vi "Replicate Core.vi"(7 "subchannel":i32, 9 "# event structures":u16=2, 10 "element (unused)":cluster{"cmd":string, "data":variant}, 11 "data in":refnum<class "EventMessengerMData.lvclass">) -> (2 "event registration refnums":refnum<event-registration>[](array[refnum]), 3 "data out":refnum<class "EventMessengerMData.lvclass">)   [LabVIEW 2019, in "Event MessengerM.lvlib" / "EventMessengerMData.lvclass"]
uses:
  EventMessengerMData.lvclass
  EventMessengerMData.lvclass/EventMessengerMData.ctl
  Event Data.ctl
  Event MessengerM.lvlib
  <vilib>/Utility/miscctls.llb/LVMapReplaceAction.ctl
panel:
  # "See note on block diagram."
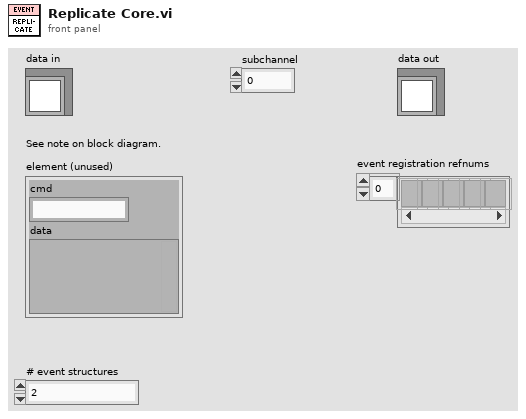
[diagram p1: front panel]
types:
  T1 = typedef "LVMapReplaceAction.ctl" = enum32{"Modify Entry only if found", "Add or Modify Entry", "Delete Entry"}
  T2 = typedef "Event MessengerM.lvlib/Event Data.ctl" = cluster{"msg":cluster{"cmd":string, "data":variant}, "valid?":bool, "last?":bool, "aborted?":bool}
  T3 = map{i32, cluster{"Write Count":u32, "Reg Refnum":u32, "aborted?":bool, "last element?":bool, "Event Refnum":refnum<user-event>}}
  T4 = cluster{"Write Count":u32, "Reg Refnum":u32, "aborted?":bool, "last element?":bool, "Event Refnum":refnum<user-event>}
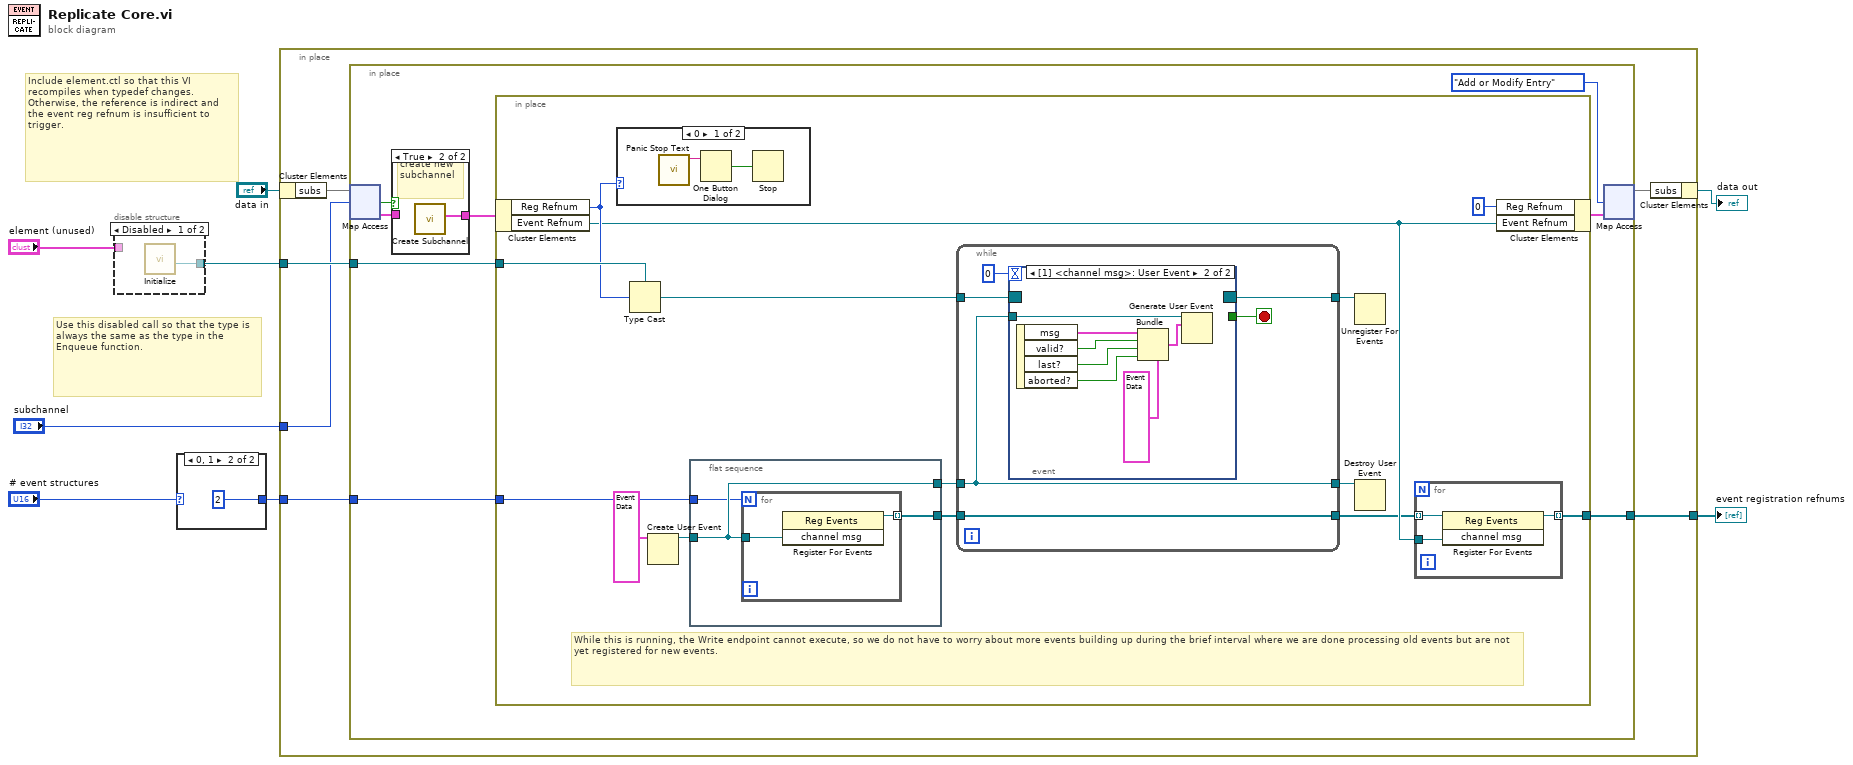
[diagram p0: block diagram]
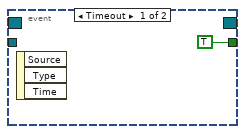
[diagram p3: hidden frame]
diagram:
  # "Include element.ctl so that this VI recompiles when typedef changes. Otherwise, the reference is indirect and the event reg refnum is insufficient to trigger."
  # "Use this disabled call so that the type is always the same as the type in the Enqueue function."
  n1 = disable-structure shown="Disabled" {
    disable-tunnel: "element (unused)" -> [_ _]
    disable-tunnel: [w9 _] -> w1
    frame Disabled {
      n2 = call "Initialize.vi"() -> ("Event Registration Refnum"=w9:refnum<event-registration>)  [unwired: 10 in, 1 out]
    }
    frame Enabled {
    }
  }
  n3 = case shown="0, 1" "# event structures" {
    selector: "# event structures" -> [w10 _]
    tunnel: [w10 u16 2] -> w5
    frame Default {
    }
    frame 0, 1 {
    }
  }
  n4 = in-place {
    in-place-border: [w17] -> w7
    in-place-border: w5 -> [w16]
    in-place-border: "subchannel" -> [w13]
    in-place-border: w1 -> [w15]
    n5 = in-place-cluster #1("data in") -> ("subs"=w14:T3)
    n6 = in-place {
      in-place-border: w15 -> [w25]
      in-place-border: [w24] -> w17
      in-place-border: w16 -> [w23]
      n7 = in-place-map #2(w14, w13) -> (w19:T4, w18:bool)  [unwired: 1 in]
      n8 = case shown="True" w18 {
        tunnel: [w26 w27] -> w20
        tunnel: w19 -> [w26 _]
        frame False {
          # "subchannel exists"
        }
        frame True {
          # "create new subchannel"
          n9 = call "Create Subchannel.vi"() -> ("subchannel"=w27:T4)  [unwired: 10 in, 1 out]
        }
      }
      n10 = in-place {
        in-place-border: w25 -> [w41]
        in-place-border: [w33] -> w24
        in-place-border: w23 -> [w30]
        # "While this is running, the Write endpoint cannot execute, so we do not have to worry about more events building up during the brief interval where we are done processing old events but are not yet registered for new events."
        n11 = in-place-cluster #3(w20) -> ("Reg Refnum"=w39:u32, "Event Refnum"=w36:refnum<user-event>)
        n12 = case shown="0" w39 {
          frame 0 {
            n13 = call "Panic Stop Text.vi"() -> ("Text"=w64:string)  [unwired: 11 in]
            n14 = One Button Dialog(message=w64) -> (true=w65:bool)  [unwired: 1 in]
            n15 = Stop(stop? (T)=w65) -> ()
          }
          frame Default {
          }
        }
        n16 = Type Cast(type=w41, x=w39) -> (*(type *) &x=w38:refnum<event-registration>)
        n17 = Create User Event(user event datatype=T2 {"msg"={"cmd"="", "data"=variant}, "valid?"=FALSE, "last?"=FALSE, "aborted?"=FALSE} ("channel msg")) -> (user event=w32:refnum<user-event>)  [unwired: 1 in, 1 out]
        n18 = flat-sequence {
          tunnel: [w44] -> w35
          tunnel: w32 -> [w43]
          tunnel: [w43] -> w31
          tunnel: w30 -> [w42]
          frame #0 {
            n19 = for {
              N: w42 -> [_]
              tunnel: w43 -> [w46]
              tunnel: [w45] -> w44 mode=indexing
              n20 = register-events(w46) -> (reference out=w45:refnum<event-registration>)  [unwired: 2 in, 1 out]
            }
          }
        }
        n21 = while {
          tunnel: w38 -> [w55]
          tunnel: [w52] -> w34
          tunnel: w35 -> [w52]
          tunnel: w31 -> [w51]
          tunnel: [w51] -> w29
          tunnel: [w50] -> w28
          stop <- w53 stop-if-true
          n22 = event shown="[1] <channel msg>: User Event" {
            selector: w55 -> [_ _]
            dyn-events: [_ _] -> w50
            timeout: 0 -> [_ _]
            tunnel: [TRUE _] -> w53
            tunnel: w51 -> [_ w63]
            event Timeout {
              n23 = event-data() -> ()  [unwired: 1 in, 3 out]
            }
            event User Event {
              n24 = event-data() -> ("msg"=w62:cluster{"cmd":string, "data":variant}, "valid?"=w61:bool, "last?"=w60:bool, "aborted?"=w59:bool)  [unwired: 1 in]
              n25 = Bundle(cluster=T2 {"msg"={"cmd"="", "data"=variant}, "valid?"=FALSE, "last?"=FALSE, "aborted?"=FALSE} ("channel msg"), "msg"=w62, "valid?"=w61, "last?"=w60, "aborted?"=w59) -> (w58:T2)
              n26 = Generate User Event(user event=w63, event data cluster=w58) -> ()  [unwired: 2 in, 2 out]
            }
          }
        }
        n27 = Unregister For Events(event registration refnum=w28) -> ()  [unwired: 1 in, 1 out]
        n28 = Destroy User Event(user event=w29) -> ()  [unwired: 1 in, 1 out]
        n29 = for {
          tunnel: w36 -> [w49]
          tunnel: [w48] -> w33 mode=indexing
          tunnel: w34 -> [w47] mode=indexing
          n30 = register-events(reference=w47, w49) -> (reference out=w48:refnum<event-registration>)  [unwired: 1 in, 1 out]
        }
        n31 = in-place-cluster #3("Reg Refnum"=u32 0, "Event Refnum"=w36) -> (w21:T4)
      }
      n32 = in-place-map #2(w21, LVMapReplaceAction."Add or Modify Entry" ("action")) -> (w12:T3)  [unwired: 2 out]
    }
    n33 = in-place-cluster #1("subs"=w12) -> (→"data out":refnum<class "EventMessengerMData.lvclass">)
  }
  "event registration refnums" <- w7
